vi "Teleop.vi"(10 "Match Info":T1={"Autonomous Elapsed Seconds"=0.0, "TeleOp Elapsed Seconds"=0.0, "Disabled Elapsed Seconds"=0.0, "Visited Autonomous"=FALSE, "Visited TeleOp"=FALSE, "Visited Disabled"=FALSE, "Autonomous Settings"={"Autonomous Style"=enum."Independent", "VI Refnum"=refnum}}, 11 "Call Context":T2) -> ()   [LabVIEW 2014]
doc: "This VI is called for each TeleOp packet received from the DS where the robot is not disabled. It is often used to read from the joysticks and update I/O or to update setpoints for timed control loops. It should complete and return within 20 milliseconds or it may miss DS packets."
uses:
  <vilib>/Rock Robotics/WPI/DriverStation/WPI_DriverStationDerivedRobotMode.ctl
  <vilib>/Rock Robotics/WPI/DriverStation/WPI_DriverStationMatch Info.ctl
  <vilib>/Rock Robotics/WPI/Joystick/WPI_JoystickGetSetRefNum.vi
  <vilib>/Rock Robotics/Network Tables/SD Write Boolean Array.vi
  <vilib>/Rock Robotics/Network Tables/SD Write Numeric Array.vi
  <vilib>/Rock Robotics/Network Tables/SD Read Boolean.vi
  <vilib>/Rock Robotics/Network Tables/SD Read Number.vi
  <vilib>/Rock Robotics/WPI/RobotDrive/WPI_RobotDriveGetSetRefNum.vi
  <vilib>/Rock Robotics/WPI/RobotDrive/WPI_RobotDriveMecanumDrive_Cartesian.vi
panel:
  out "Throttle":dbl
  out "Sample Slider 0":dbl(slide) scale=0.0..5.0
  out "Sample Boolean 1":bool
  out "Sample Boolean 0":bool
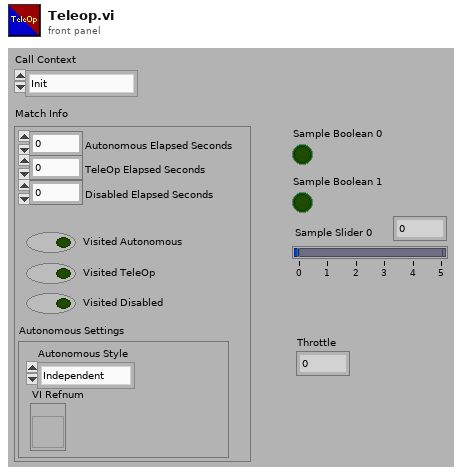
[diagram p1: front panel]
types:
  T1 = typedef "WPI_DriverStationMatch Info.ctl" = cluster{"Autonomous Elapsed Seconds":dbl, "TeleOp Elapsed Seconds":dbl, "Disabled Elapsed Seconds":dbl, "Visited Autonomous":bool, "Visited TeleOp":bool, "Visited Disabled":bool, "Autonomous Settings":cluster{"Autonomous Style":enum16{"Iterative", "Independent"}, "VI Refnum":refnum<vi>}}
  T2 = typedef "WPI_DriverStationDerivedRobotMode.ctl" = enum16{"Init", "Execute", "Stop"}
  T3 = typedef "WPI_RobotDriveDevRef.ctl" = cluster{"DevStatus":errorcluster, "Motors[]":T4[], "Square Inputs":bool, "Max Output":dbl}
  T4 = typedef "WPI_MotorControlDeviceRef.ctl" = cluster{"DeviceStatus":errorcluster, "Type":T5, "PWM":cluster{"Controller":T6, "PWM Channel":T7, "DeadBand":T8}, "CAN":cluster{"Device Number":u8, "Control Mode":T9, "Semaphore":T10, "Max Vout":dbl, "TalonSRX Control Mode":T11}, "Invert":bool, "TransformRef":T12, "InvTransformRef":T12}
  T5 = typedef "WPI_MotorControlType.ctl" = enum16{"PWM", "CAN", "CANTalonSRX"}
  T6 = typedef "FPGA_TypedefDigitalModule.ctl" = enum16{"Controller 1"}
  T7 = typedef "FPGA_DIOPWMChannel.ctl" = enum8{"PWM 0", "PWM 1", "PWM 2", "PWM 3", "PWM 4", "PWM 5", "PWM 6", "PWM 7", "PWM 8", "PWM 9", "PWM MXP 0", "PWM MXP 1", "PWM MXP 2", "PWM MXP 3", "PWM MXP 4", "PWM MXP 5", "PWM MXP 6", "PWM MXP 7", "PWM MXP 8", "PWM MXP 9", "Invalid"}
  T8 = typedef "WPI_PWMDeadband.ctl" = cluster{"Name":string, "maxPositivePwm":i32, "minPositivePwm":i32, "centerPwm":i32, "maxNegativePwm":i32, "minNegativePwm":i32, "angularRange":u16}
  T9 = typedef "WPI_CANJaguar_ControlMode.ctl" = enum8{"Percent VBus", "Current", "Speed", "Position", "Voltage"}
  T10 = typedef "Semaphore RefNum" = refnum<k1>
  T11 = typedef "WPI_CANTalonSRX_APIControlMode.ctl" = enum8{"Percent VBus", "Speed", "Position", "Slave", "Unchanged / Invalid"}
  T12 = typedef "WPI_PWMTransform_ConPane.ctl" = refnum<vi>
  T13 = typedef "WPI_JoystickDevRef.ctl" = cluster{"Device":T14}
  T14 = typedef "WPI_JoystickDeviceEnum.ctl" = enum16{"USB 0", "USB 1", "USB 2", "USB 3", "USB 4", "USB 5"}
  T15 = typedef "WPI_ServoDeviceRef.ctl" = cluster{"DeviceStatus":errorcluster, "Controller":T6, "PWM Channel":T7, "DeadBand":T8}
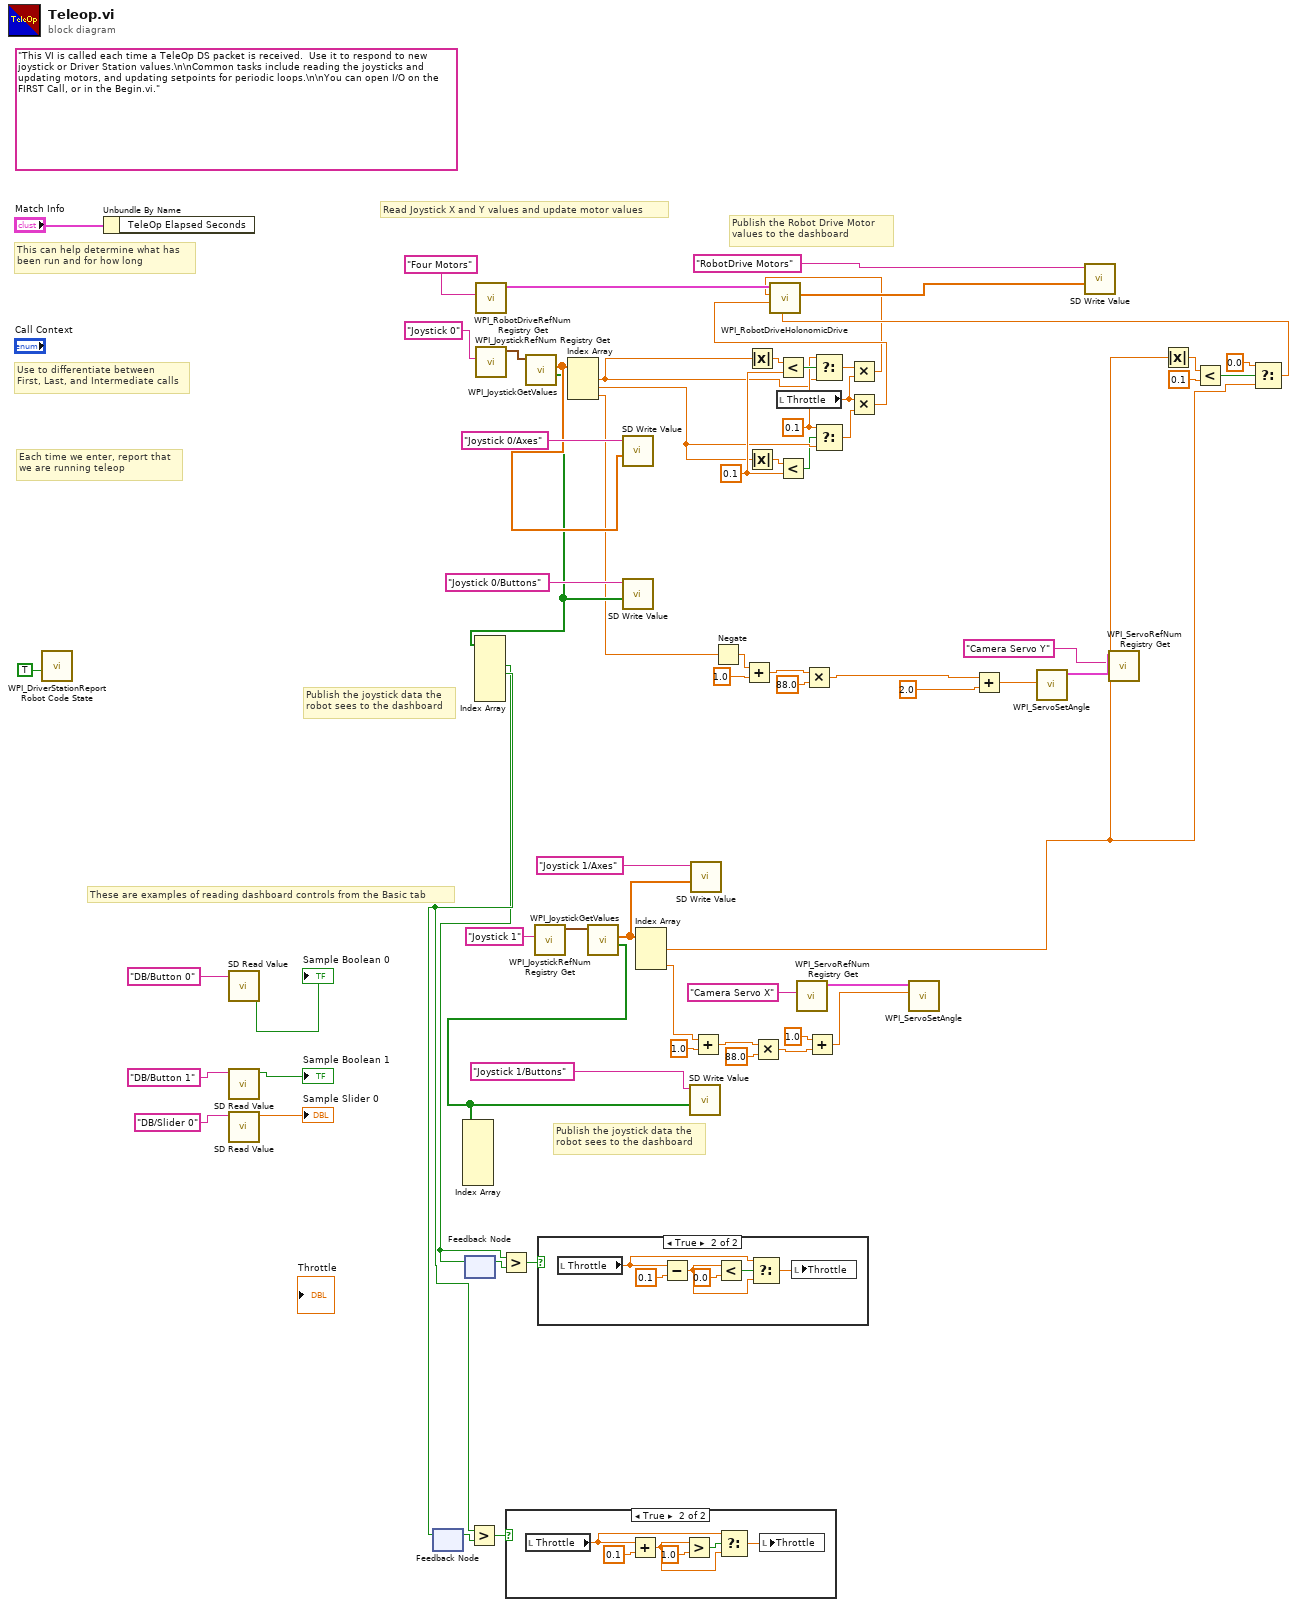
[diagram p0: block diagram]
diagram:
  w25 = 0.1
  w30 = 0.1
  (unwired) "This VI is called each time a TeleOp DS packet is received.  Use it to respond to new joystick or Driver Station values.\n\nCommon tasks include reading the joysticks and updating motors, and updating setpoints for periodic loops.\n\nYou can open I/O on the FIRST Call, or in the Begin.vi."
  # "Publish the joystick data the\nrobot sees to the dashboard"
  # "These are examples of reading dashboard controls from the Basic tab"
  # "Publish the Robot Drive Motor\nvalues to the dashboard"
  # "Publish the joystick data the\nrobot sees to the dashboard"
  # "Each time we enter, report that\nwe are running teleop"
  # "Use to differentiate between\nFirst, Last, and Intermediate calls"
  # "This can help determine what has\nbeen run and for how long"
  # "Read Joystick X and Y values and update motor values"
  n1 = call <vilib>:"WPI_DriverStationReport Robot Code State.vi"("TeleOp"=TRUE ("Autonomous")) -> ()  [unwired: 10 in, 1 out]
  n2 = Unbundle By Name("Match Info") -> ()  [unwired: 1 out]
  n3 = call-poly <vilib>:"SD Read Value.vi"("Name"="DB/Button 0" ("refnum name")) -> ("Boolean"=→"Sample Boolean 0":bool)  [unwired: 8 in, 2 out]
  n4 = call-poly <vilib>:"SD Read Value.vi"("Name"="DB/Button 1" ("refnum name")) -> ("Boolean"=→"Sample Boolean 1":bool)  [unwired: 8 in, 2 out]
  n5 = call-poly <vilib>:"SD Read Value.vi"("Name"="DB/Slider 0" ("refnum name")) -> ("Numeric"=→"Sample Slider 0":dbl)  [unwired: 8 in, 2 out]
  n6 = feedback #1() -> (w10:bool)  [unwired: 1 in]
  n7 = feedback #2() -> (w6:bool)  [unwired: 1 in]
  n8 = call <vilib>:"WPI_RobotDriveRefNum Registry Get.vi"("refnum name"="Four Motors") -> ("RobotDriveDevRef"=w66:T3)  [unwired: 1 in, 9 out]
  n9 = call <vilib>:"WPI_JoystickRefNum Registry Get.vi"("refnum name"="Joystick 0") -> ("JoystickDevRef"=w64:T13)  [unwired: 1 in, 9 out]
  n10 = call <vilib>:"WPI_JoystickGetValues.vi"("JoystickDevRef"=w64) -> ("Buttons"=w44:bool[], "Axes"=w52:dbl[])  [unwired: 6 in, 3 out]
  n11 = Index Array(array=w44) -> (element #2=w8:bool, element #3=w9:bool)  [unwired: 6 in, 4 out]
  n12 = feedback-in #1(w9) -> ()
  n13 = feedback-in #2(w8) -> ()
  n14 = Greater?(x=w9, y=w10) -> (0:w11:bool)
  n15 = Greater?(x=w8, y=w6) -> (0:w7:bool)
  n16 = case shown="True" w11 {
    frame False {
    }
    frame True {
      n17 = local read "Throttle"() -> (w71:dbl)
      n18 = Add(x=w71, y=0.1) -> (x+y=w70:dbl)
      n19 = Greater?(x=w70, y=1.0) -> (0:w72:bool)
      n20 = Select(t=w71, s=w72, f=w70) -> (s? t:f=w69:dbl)
      n21 = local write "Throttle"(w69) -> ()
    }
  }
  n22 = call <vilib>:"WPI_JoystickRefNum Registry Get.vi"("refnum name"="Joystick 1") -> ("JoystickDevRef"=w50:T13)  [unwired: 1 in, 9 out]
  n23 = case shown="True" w7 {
    frame False {
    }
    frame True {
      n24 = local read "Throttle"() -> (w79:dbl)
      n25 = Subtract(x=w79, y=0.1) -> (x-y=w76:dbl)
      n26 = Less?(x=w76, y=0.0) -> (x < y?=w77:bool)
      n27 = Select(t=w79, s=w77, f=w76) -> (s? t:f=w78:dbl)
      n28 = local write "Throttle"(w78) -> ()
    }
  }
  n29 = Index Array(array=w52) -> (element #1=w18:dbl, element #2=w29:dbl, element #3=w17:dbl)  [unwired: 3 in]
  n30 = call <vilib>:"WPI_JoystickGetValues.vi"("JoystickDevRef"=w50) -> ("Buttons"=w45:bool[], "Axes"=w47:dbl[])  [unwired: 6 in, 3 out]
  n31 = Index Array(array=w45) -> ()  [unwired: 6 in, 6 out]
  n32 = call-poly <vilib>:"SD Write Value.vi"("Numeric Array"=w52, "Name"="Joystick 0/Axes") -> ()  [unwired: 8 in, 2 out]
  n33 = call-poly <vilib>:"SD Write Value.vi"("Boolean Array"=w44, "Name"="Joystick 0/Buttons") -> ()  [unwired: 8 in, 2 out]
  n34 = Index Array(array=w47) -> (element #1=w20:dbl, element #3=w13:dbl)  [unwired: 3 in, 1 out]
  n35 = call-poly <vilib>:"SD Write Value.vi"("Boolean Array"=w45, "Name"="Joystick 1/Buttons") -> ()  [unwired: 8 in, 2 out]
  n36 = call-poly <vilib>:"SD Write Value.vi"("Numeric Array"=w47, "Name"="Joystick 1/Axes") -> ()  [unwired: 8 in, 2 out]
  n37 = Add(x=w13, y=1.0) -> (x+y=w38:dbl)
  n38 = Negate(x=w17) -> (-x=w16:dbl)
  n39 = Add(x=w16, y=1.0) -> (x+y=w15:dbl)
  n40 = Absolute Value(x=w18) -> (abs(x)=w27:dbl)
  n41 = Absolute Value(x=w29) -> (abs(x)=w28:dbl)
  n42 = Multiply(x=w38, y=88.0) -> (x*y=w34:dbl)
  n43 = local read "Throttle"() -> (w5:dbl)
  n44 = Less?(x=w27, y=w30) -> (x < y?=w31:bool)
  n45 = Less?(x=w28, y=w30) -> (x < y?=w26:bool)
  n46 = call <vilib>:"WPI_ServoRefNum Registry Get.vi"("refnum name"="Camera Servo X") -> ("ServoDeviceRef"=w46:T15)  [unwired: 9 in, 1 out]
  n47 = Multiply(x=w15, y=88.0) -> (x*y=w36:dbl)
  n48 = Add(x=1.0, y=w34) -> (x+y=w32:dbl)
  n49 = Select(t=w25, s=w31, f=w18) -> (s? t:f=w2:dbl)
  n50 = Select(t=w25, s=w26, f=w29) -> (s? t:f=w4:dbl)
  n51 = Multiply(x=w2, y=w5) -> (x*y=w1:dbl)
  n52 = Multiply(x=w5, y=w4) -> (x*y=w3:dbl)
  n53 = call <vilib>:"WPI_ServoSetAngle.vi"("Angle"=w32, "ServoDeviceRef"=w46) -> ()  [unwired: 8 in, 2 out]
  n54 = Add(x=w36, y=2.0) -> (x+y=w14:dbl)
  n55 = call <vilib>:"WPI_ServoRefNum Registry Get.vi"("refnum name"="Camera Servo Y") -> ("ServoDeviceRef"=w43:T15)  [unwired: 9 in, 1 out]
  n56 = call <vilib>:"WPI_ServoSetAngle.vi"("Angle"=w14, "ServoDeviceRef"=w43) -> ()  [unwired: 8 in, 2 out]
  n57 = Absolute Value(x=w20) -> (abs(x)=w22:dbl)
  n58 = Less?(x=w22, y=0.1) -> (x < y?=w24:bool)
  n59 = Select(t=0.0, s=w24, f=w20) -> (s? t:f=w19:dbl)
  n60 = call-poly <vilib>:"WPI_RobotDriveHolonomicDrive.vi"("Rotation"=w19, "Y"=w3, "X"=w1, "RobotDriveDevRef"=w66) -> ("Motor Values"=w53:dbl[])  [unwired: 5 in, 2 out]
  n61 = call-poly <vilib>:"SD Write Value.vi"("Numeric Array"=w53, "Name"="RobotDrive Motors") -> ()  [unwired: 8 in, 2 out]
